vi "R1GetOtherConstants.vi"(7 "LabVIEW Web Service Request":refnum<class "Web Request.lvclass">, 10 "cRIONo":i32=1, 11 "ReactorNo":i32=1) -> (3 "Array":string[](array[string]))   [LabVIEW 2016]
uses:
  <vilib>/wsapi/Web Request.lvclass
  <resource>/objmgr/ni.var.rc
panel:
  # "Use the Web Service Request input terminal to call the VIs on the Web Services palette. Do not remove it from the connector pane unless you don't need access to the palette."
  # "Each additional control wired to the connector pane will be available as an input in the URL. To include an indicator in terminal-mode output (the default setting), it must also be wired to the connector pane."
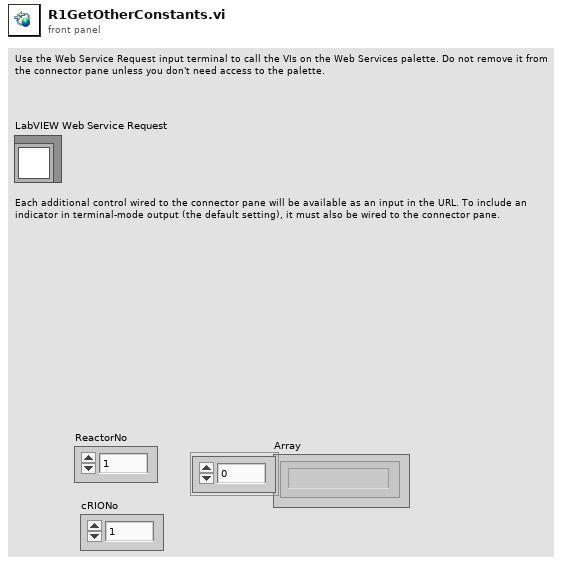
[diagram p1: front panel]
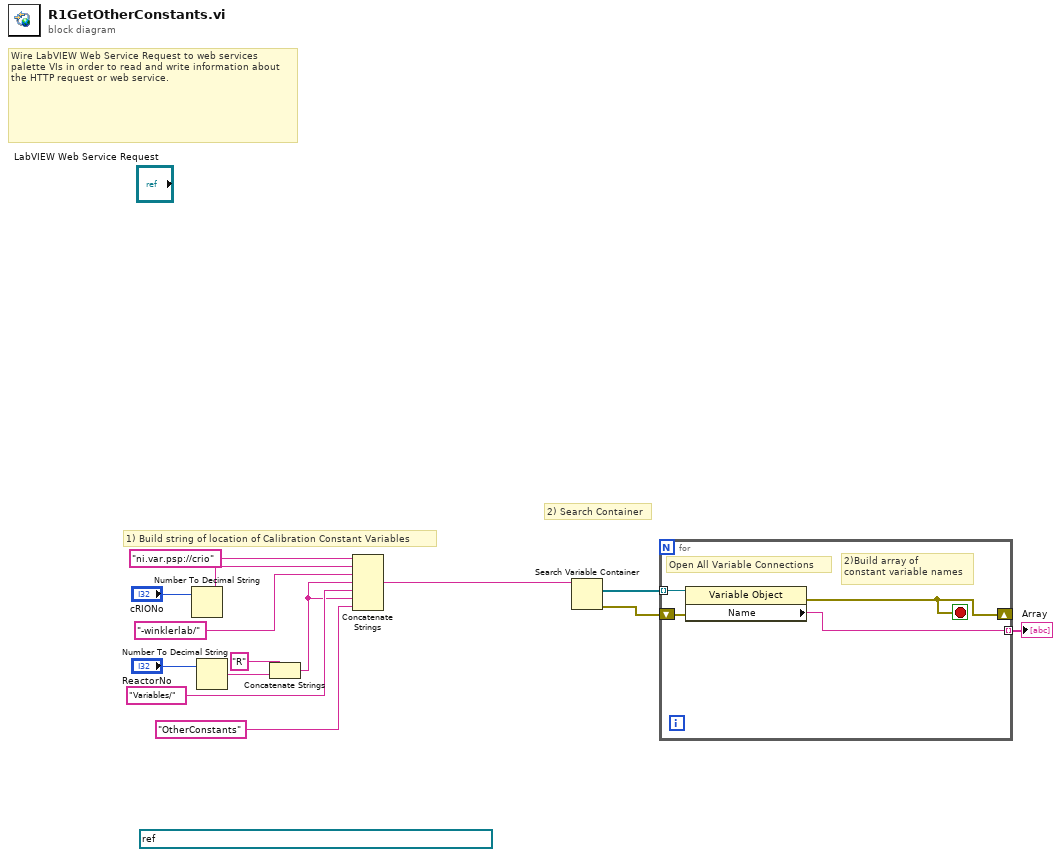
[diagram p0: block diagram]
diagram:
  (unwired) refnum<k21> "ni.var.psp://cRIO1-WinklerLab/R1Variables/R1OtherConstants" ("shared variable refnum in")
  # "2) Search Container"
  # "1) Build string of location of Calibration Constant Variables"
  # "Wire LabVIEW Web Service Request to web services palette VIs in order to read and write information about the HTTP request or web service."
  n1 = Number To Decimal String(number="cRIONo") -> (decimal integer string=w9:string)  [unwired: 1 in]
  n2 = Number To Decimal String(number="ReactorNo") -> (decimal integer string=w12:string)  [unwired: 1 in]
  n3 = Concatenate Strings("R" ("string"), w12) -> (w6:string)
  n4 = Concatenate Strings("ni.var.psp://crio" ("string"), w9, "-winklerlab/" ("string"), w6, "Variables/" ("string"), w6, "OtherConstants" ("string")) -> (w1:string)
  n5 = Search Variable Container(11:w1) -> (0:w5:errorcluster, 2:w3:refnum<k21>[])  [unwired: 5 in, 1 out]
  n6 = for {
    shift-right: [w16] -> _
    shift-left: w5 -> [w18]
    tunnel: [w17] -> w4 mode=indexing
    tunnel: w3 -> [w15] mode=indexing
    stop <- w16 stop-if-true
    # "2)Build array of \nconstant variable names"
    # "Open All Variable Connections"
    n7 = property class="Variable Object"(reference=w15, error in=w18) -> (error out=w16:errorcluster, "Name"=w17:string)  [unwired: 1 out]
  }
  "Array" <- w4
